vi "Log_Apontamento.vi"() -> ()   [LabVIEW 2018]
uses:
  Global_Telescopio.vi
panel:
  out "Comando":string
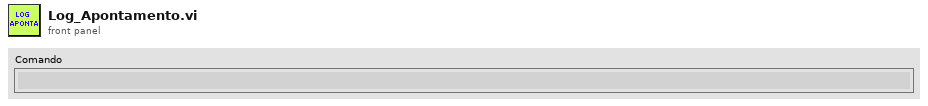
[diagram p1: front panel]
types:
  T1 = enum16{"open", "open or create", "create or replace", "create"}
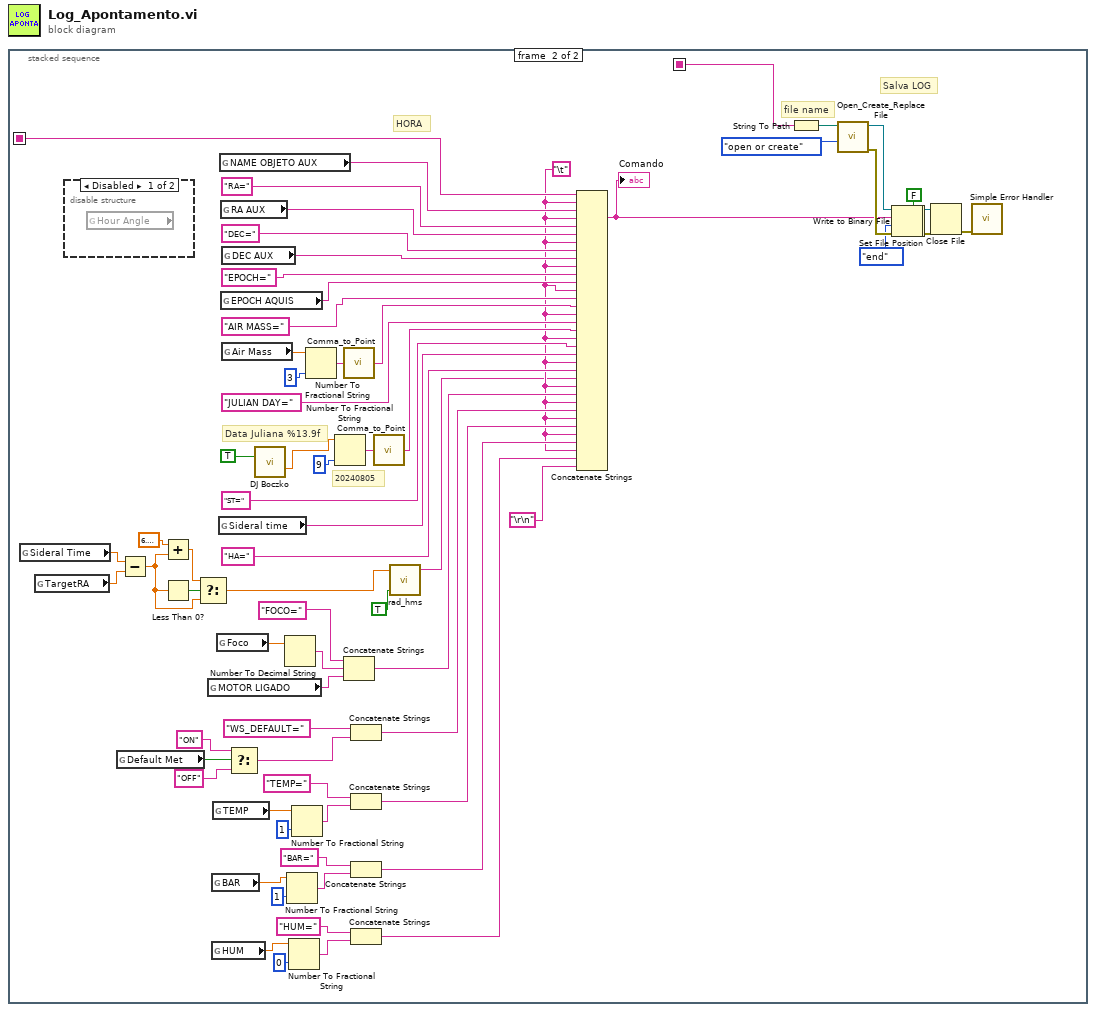
[diagram p0: block diagram]
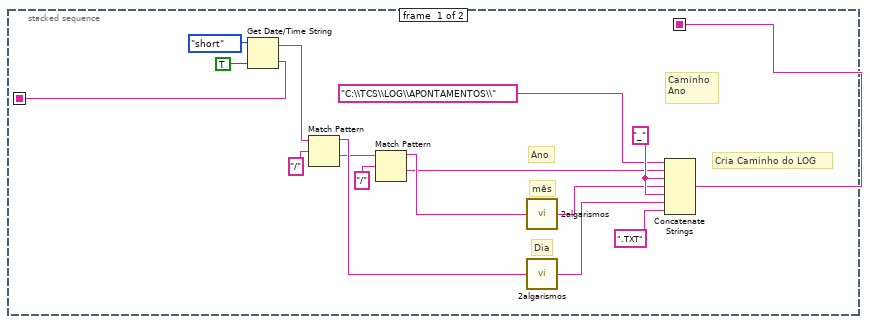
[diagram p2: hidden frame]
diagram:
  n1 = stacked-sequence {
    seq-local: [w1 _] -> [_ w78]
    seq-local: [w6 _] -> [_ w88]
    frame #0 {
      w15 = "_"
      # "Cria Caminho do LOG"
      # "Caminho\nAno"
      # "Ano"
      # "mês"
      # "Dia"
      n2 = Get Date/Time String(date format (0)=enum16{"short", "long", "abbreviated"}."short", want seconds? (F)=TRUE) -> (date string=w14:string, time string=w6:string)  [unwired: 1 in]
      n3 = Match Pattern(string=w14, regular expression="/") -> (before substring=w16:string, after substring=w11:string)  [unwired: 1 in, 2 out]
      n4 = Match Pattern(string=w11, regular expression="/") -> (before substring=w10:string, after substring=w9:string)  [unwired: 1 in, 2 out]
      n5 = call "2algarismos.vi"("entrada"=w10) -> ("saida"=w4:string)
      n6 = call "2algarismos.vi"("entrada"=w16) -> ("saida"=w3:string)
      n7 = Concatenate Strings("C:\\TCS\\LOG\\APONTAMENTOS\\" ("SOMENTE DIRETORIO"), w9, w15, w4, w15, w3, ".TXT" ("regular expression")) -> (w1:string)
    }
    frame #1 {
      w32 = "\t"
      # "20240805"
      # "Data Juliana %13.9f"
      # "HORA"
      # "Salva LOG"
      # "file name"
      n8 = global read "Global_Telescopio.vi" "Sideral Time"() -> (w25:dbl)
      n9 = global read "Global_Telescopio.vi" "TargetRA"() -> (w26:dbl)
      n10 = disable-structure shown="Disabled" {
        frame Disabled {
          n11 = global read "Global_Telescopio.vi" "Hour Angle"() -> ()  [unwired: 1 out]
        }
        frame Enabled {
        }
      }
      n12 = global read "Global_Telescopio.vi" "Default Met"() -> (w20:bool)
      n13 = Subtract(x=w25, y=w26) -> (x-y=w24:dbl)
      n14 = Add(x=6.283185307179586, y=w24) -> (x+y=w28:dbl)
      n15 = Less Than 0?(x=w24) -> (x < 0?=w27:bool)
      n16 = Select(t=w28, s=w27, f=w24) -> (s? t:f=w22:dbl)
      n17 = global read "Global_Telescopio.vi" "MOTOR LIGADO"() -> (w38:string)
      n18 = global read "Global_Telescopio.vi" "BAR"() -> (w43:dbl)
      n19 = global read "Global_Telescopio.vi" "HUM"() -> (w44:dbl)
      n20 = global read "Global_Telescopio.vi" "TEMP"() -> (w39:dbl)
      n21 = global read "Global_Telescopio.vi" "Foco"() -> (w52:dbl)
      n22 = global read "Global_Telescopio.vi" "Sideral time"() -> (w55:string)
      n23 = global read "Global_Telescopio.vi" "NAME OBJETO AUX"() -> (w74:string)
      n24 = global read "Global_Telescopio.vi" "RA AUX"() -> (w72:string)
      n25 = global read "Global_Telescopio.vi" "EPOCH AQUIS"() -> (w68:string)
      n26 = global read "Global_Telescopio.vi" "DEC AUX"() -> (w70:string)
      n27 = global read "Global_Telescopio.vi" "Air Mass"() -> (w65:dbl)
      n28 = Select(t="ON", s=w20, f="OFF") -> (s? t:f=w17:string)
      n29 = call "DJ Boczko.vi"("TRUE = Hora Local\nFALSE = UT"=TRUE ("TRUE = Hora Local\nFALSE = UT")) -> ("Dia Juliano"=w61:dbl)  [unwired: 6 in, 8 out]
      n30 = Number To Decimal String(number=w52) -> (decimal integer string=w53:string)  [unwired: 1 in]
      n31 = Number To Fractional String(number=w43, precision (6)=i16 1) -> (F-format string=w50:string)  [unwired: 2 in]
      n32 = Number To Fractional String(number=w44, precision (6)=i16 0) -> (F-format string=w51:string)  [unwired: 2 in]
      n33 = Number To Fractional String(number=w39, precision (6)=i16 1) -> (F-format string=w48:string)  [unwired: 2 in]
      n34 = Number To Fractional String(number=w65, precision (6)=i16 3) -> (F-format string=w67:string)  [unwired: 2 in]
      n35 = Number To Fractional String(number=w61, precision (6)=i16 9) -> (F-format string=w62:string)  [unwired: 2 in]
      n36 = call "Comma_to_Point.vi"("Lat_A"=w67) -> ("Saída"=w63:string)
      n37 = Concatenate Strings("FOCO=", w53, w38) -> (w36:string)
      n38 = Concatenate Strings("WS_DEFAULT=" ("string"), w17) -> (w35:string)
      n39 = Concatenate Strings("TEMP=" ("string"), w48) -> (w34:string)
      n40 = Concatenate Strings("BAR=" ("string"), w50) -> (w33:string)
      n41 = Concatenate Strings("HUM=" ("string"), w51) -> (w31:string)
      n42 = call "Comma_to_Point.vi"("Lat_A"=w62) -> ("Saída"=w57:string)
      n43 = call "rad_hms.vi"("TRUE=HORA\nFALSE=GRAU"=TRUE ("TRUE=HORA\nFALSE=GRAU"), "Radiano"=w22) -> ("Hora/Graus Texto Decimal"=w21:string)  [unwired: 3 in]
      n44 = Concatenate Strings(w88, w32, w74, w32, "RA=", w72, w32, "DEC=", w70, w32, "EPOCH=", w68, w32, "AIR MASS=", w63, w32, "JULIAN DAY=", w57, w32, "ST=", w55, w32, "HA=", w21, w32, w36, w32, w35, w32, w34, w32, w33, w32, w31, "\r\n") -> (w79:string)
      "Comando" <- w79
      n45 = String To Path(string=w78) -> (path=w80:path)
      n46 = call <vilib>:"Open_Create_Replace File.vi"("function (open:0)"=T1."open or create", "file path"=w80) -> ("error out"=w83:errorcluster, "refnum"=w86:refnum<file>)  [unwired: 6 in, 2 out]
      n47 = Set File Position(refnum=w86, from (0:start)=enum16{"start", "end", "current"}."end" ("pos mode (0:2)"), error in=w83) -> (refnum out=w77:refnum<file>, error out=w76:errorcluster)  [unwired: 1 in]
      n48 = Write to Binary File(file (use dialog)=w77, data=w79, error in=w76, 5:FALSE ("prepend array or string size? (T)")) -> (refnum out=w85:refnum<file>, error out=w84:errorcluster)  [unwired: 2 in, 1 out]
      n49 = Close File(refnum=w85, error in=w84) -> (error out=w87:errorcluster)  [unwired: 1 out]
      n50 = call <vilib>:"Simple Error Handler.vi"("error in (no error)"=w87) -> ()  [unwired: 4 in, 5 out]
    }
  }
